vi "Post (U64 Array).vi"(6 "timestamp in":timestamp, 7 "PV name":string, 8 "error in (no error)":errorcluster, 10 "value in":u64[](array[numeric]), 11 "Server in":refnum<class "Server.lvclass">) -> (0 "error out":errorcluster, 2 "value out":u64[](array[numeric]), 3 "Server out":refnum<class "Server.lvclass">, 4 "timestamp out":timestamp)   [LabVIEW 2020, in "PV Access.lvlib" / "PVA Server.lvlib" / "Server.lvclass"]
uses:
  Server.lvclass
  Server.lvclass/Server.ctl
  25a0afa2-78cc-4e41-9cb9-729b0faefda4.vi
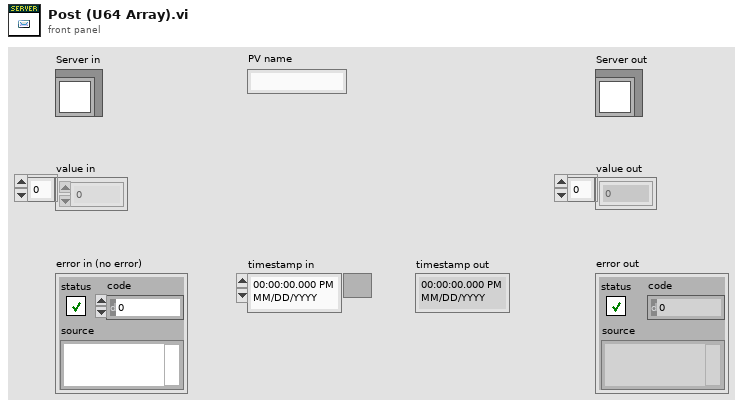
[diagram p1: front panel]
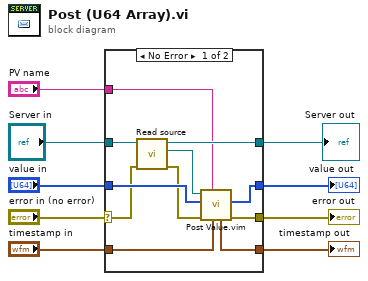
[diagram p0: block diagram]
diagram:
  n1 = case shown="No Error" "error in (no error)" {
    selector: "error in (no error)" -> [w13 w24]
    tunnel: [w14 w24] -> w3
    tunnel: [w19 w23] -> w1
    tunnel: "Server in" -> [w20 w23]
    tunnel: "PV name" -> [w15 _]
    tunnel: "value in" -> [w17 w22]
    tunnel: [w18 w22] -> w4
    tunnel: "timestamp in" -> [w11 w21]
    tunnel: [w10 w21] -> w2
    frame No Error {
      n2 = call "Read source.vi"("error in (no error)"=w13, "Server in"=w20) -> ("error out"=w12:errorcluster, "Source"=w16:refnum<class "Source.lvclass">, "Server out"=w19:refnum<class "Server.lvclass">)  [unwired: 7 in]
      n3 = call "Post Value.vim"("timestamp in"=w11, "PV name"=w15, "error in"=w12, "value in"=w17, "Source in"=w16) -> ("error out"=w14:errorcluster, "value out"=w18:u64[], "timestamp out"=w10:timestamp)  [unwired: 3 in, 1 out]
    }
    frame Error {
    }
  }
  "error out" <- w3
  "Server out" <- w1
  "value out" <- w4
  "timestamp out" <- w2
